vi "SpecAn Capture Screenshot.vi"(0 "VISA In":refnum<visa-resource-name>, 5 "Error In":errorcluster, 6 "Full Screen":bool, 7 "Secured View":bool, 9 "Save Image?":bool) -> (13 "image size":cluster{"Width":u32, "Height":u32}, 14 "VISA Out":refnum<visa-resource-name>, 15 "image data":T1, 16 "Pic":picture, 18 "GIF_PATH":path, 19 "Error Out":errorcluster)   [LabVIEW 2015]
uses:
  <vilib>/picture/picture.llb/imagedata.ctl
  Controls/FGV Action SpecAn Model.ctl
  <vilib>/wsapi/NI_WebServices.lvlib
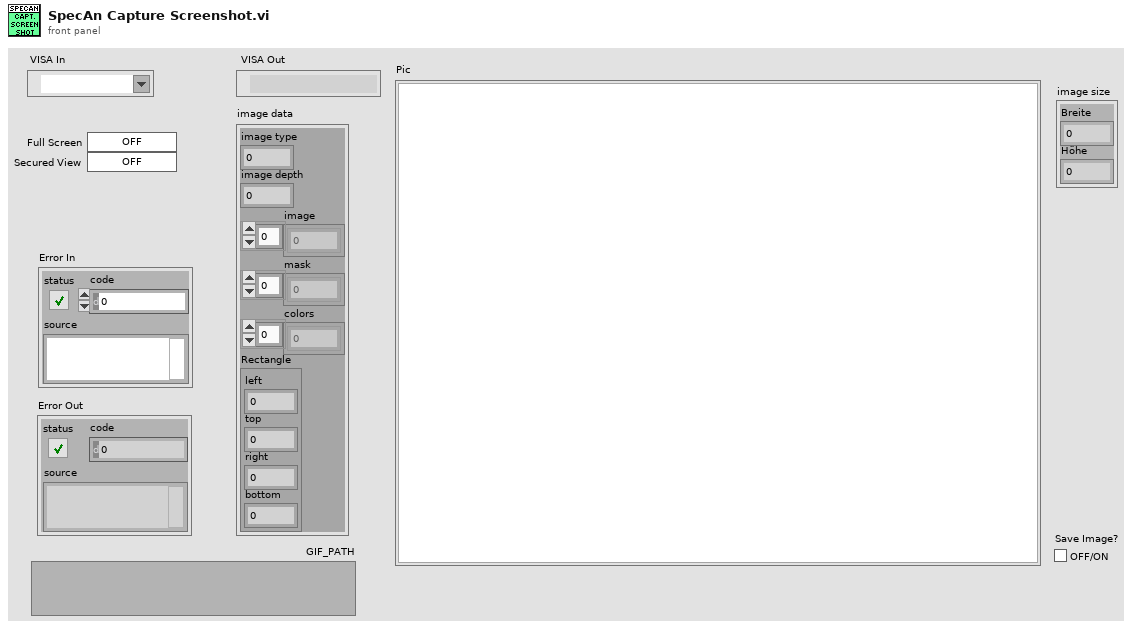
[diagram p1: front panel]
types:
  T1 = typedef "imagedata.ctl" = cluster{"image type":i32, "image depth":i32, "image":u8[], "mask":u8[], "colors":u32[], "Rectangle":cluster{"left":i16, "top":i16, "right":i16, "bottom":i16}}
  T2 = typedef "FGV Action SpecAn Model.ctl" = enum16{"Get", "Set"}
  T3 = typedef "SpecAn Model.ctl" = enum16{"E4440", "N9030"}
  T4 = enum16{"big-endian, network order", "native, host order", "little-endian"}
  T5 = cluster{"left":i16, "top":i16, "right":i16, "bottom":i16}
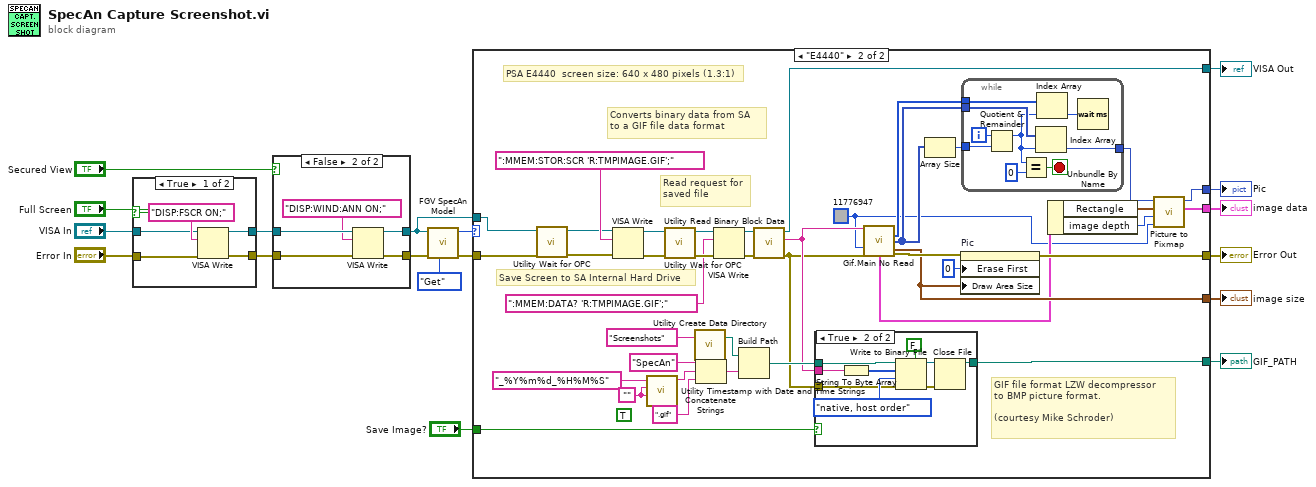
[diagram p0: block diagram]
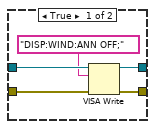
[diagram p2: hidden frame]
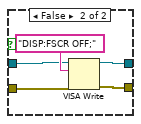
[diagram p3: hidden frame]
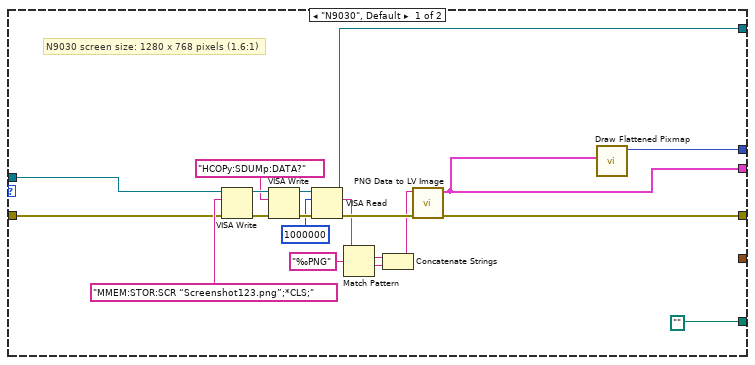
[diagram p4: hidden frame]
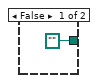
[diagram p5: hidden frame]
diagram:
  n1 = case shown="True" "Full Screen" {
    tunnel: [w22 w27] -> w5
    tunnel: [w21 w26] -> w9
    tunnel: "Error In" -> [w19 w25]
    tunnel: "VISA In" -> [w20 w24]
    frame True {
      n2 = VISA Write(VISA resource name=w20, write buffer="DISP:FSCR ON;", error in (no error)=w19) -> (VISA resource name out=w22:refnum<visa-resource-name>, error out=w21:errorcluster)  [unwired: 1 out]
    }
    frame False {
      n3 = VISA Write(VISA resource name=w24, write buffer="DISP:FSCR OFF;", error in (no error)=w25) -> (VISA resource name out=w27:refnum<visa-resource-name>, error out=w26:errorcluster)  [unwired: 1 out]
    }
  }
  n4 = case shown="False" "Secured View" {
    tunnel: w5 -> [w33 w38]
    tunnel: [w32 w37] -> w3
    tunnel: [w31 w36] -> w4
    tunnel: w9 -> [w29 w34]
    frame True {
      n5 = VISA Write(VISA resource name=w33, write buffer="DISP:WIND:ANN OFF;", error in (no error)=w29) -> (VISA resource name out=w32:refnum<visa-resource-name>, error out=w31:errorcluster)  [unwired: 1 out]
    }
    frame False {
      n6 = VISA Write(VISA resource name=w38, write buffer="DISP:WIND:ANN ON;", error in (no error)=w34) -> (VISA resource name out=w37:refnum<visa-resource-name>, error out=w36:errorcluster)  [unwired: 1 out]
    }
  }
  n7 = call "FGV SpecAn Model.vi"("Action"=FGV_Action_SpecAn_Model."Get", "Error In"=w4, "VISA In"=w3) -> ("Error Out"=w2:errorcluster, "SA Model"=w16:T3)  [unwired: 4 in]
  n8 = case shown="\"E4440\"" w16 {
    tunnel: [w39 w76] -> w14
    tunnel: w2 -> [w48 w60]
    tunnel: w3 -> [w47 w61]
    tunnel: [w46 w91] -> w18
    tunnel: [w43 w63] -> w15
    tunnel: [w42 w62] -> w13
    tunnel: [path "" w71] -> w12
    tunnel: [_ w69] -> w11
    tunnel: "Save Image?" -> [_ w59]
    frame "N9030", Default {
      # "N9030 screen size: 1280 x 768 pixels (1.6:1)"
      n9 = VISA Write(VISA resource name=w47, write buffer="MMEM:STOR:SCR “Screenshot123.png”;*CLS;", error in (no error)=w48) -> (VISA resource name out=w56:refnum<visa-resource-name>, error out=w57:errorcluster)  [unwired: 1 out]
      n10 = VISA Write(VISA resource name=w56, write buffer="HCOPy:SDUMp:DATA?", error in (no error)=w57) -> (VISA resource name out=w53:refnum<visa-resource-name>, error out=w54:errorcluster)  [unwired: 1 out]
      n11 = VISA Read(VISA resource name=w53, byte count=u32 1000000, error in (no error)=w54) -> (VISA resource name out=w46:refnum<visa-resource-name>, read buffer=w44:string, error out=w45:errorcluster)  [unwired: 1 out]
      n12 = Match Pattern(string=w44, regular expression="‰PNG") -> (match substring=w50:string, after substring=w49:string)  [unwired: 1 in, 2 out]
      n13 = Concatenate Strings(w50, w49) -> (w41:string)
      n14 = call <vilib>:"PNG Data to LV Image.vi"("error in (no error)"=w45, "png data"=w41) -> ("error out"=w39:errorcluster, "image data"=w43:T1)  [unwired: 8 in]
      n15 = call <vilib>:"Draw Flattened Pixmap.vi"("image data"=w43) -> ("new picture"=w42:picture)  [unwired: 8 in]
    }
    frame "E4440" {
      (unwired) TRUE
      w82 = ""
      w65 = u32 11776947 ("bgcolor")
      # "PSA E4440  screen size: 640 x 480 pixels (1.3:1)"
      # "GIF file format LZW decompressor\nto BMP picture format.\n\n(courtesy Mike Schroder)"
      # "Converts binary data from SA\nto a GIF file data format"
      # "Read request for\nsaved file"
      # "Save Screen to SA Internal Hard Drive"
      n16 = call "Utility Wait for OPC.vi"("error in (no error)"=w60, "VISA resource name"=w61) -> ("error out"=w89:errorcluster, "VISA resource name out"=w88:refnum<visa-resource-name>)  [unwired: 8 in]
      n17 = VISA Write(VISA resource name=w88, write buffer=":MMEM:STOR:SCR 'R:TMPIMAGE.GIF';", error in (no error)=w89) -> (VISA resource name out=w95:refnum<visa-resource-name>, error out=w93:errorcluster)  [unwired: 1 out]
      n18 = call "Utility Timestamp with Date and Time Strings.vi"("Delimiter (Time)"=w82, "Delimiter (Date)"=w82, "Timestamp Format String"="_%Y%m%d_%H%M%S" ("time format string (%c)")) -> ("Timestamp String"=w80:string)  [unwired: 6 in, 2 out]
      n19 = call "Utility Wait for OPC.vi"("error in (no error)"=w93, "VISA resource name"=w95) -> ("error out"=w94:errorcluster, "VISA resource name out"=w96:refnum<visa-resource-name>)  [unwired: 8 in]
      n20 = call "Utility Create Data Directory.vi"("Folder Name"="Screenshots") -> ("Path"=w84:path)  [unwired: 2 in]
      n21 = Concatenate Strings("SpecAn" ("File Name"), w80, ".gif" ("string")) -> (w79:string)
      n22 = VISA Write(VISA resource name=w96, write buffer=":MMEM:DATA? 'R:TMPIMAGE.GIF';", error in (no error)=w94) -> (VISA resource name out=w98:refnum<visa-resource-name>, error out=w97:errorcluster)  [unwired: 1 out]
      n23 = Build Path(base path=w84, name or relative path=w79) -> (appended path=w77:path)
      n24 = call "Utility Read Binary Block Data.vi"("Error In"=w97, "VISA In"=w98) -> ("Error Out"=w66:errorcluster, "Data"=w74:string, "VISA Out"=w91:refnum<visa-resource-name>)  [unwired: 5 in]
      n25 = case shown="True" w59 {
        tunnel: w77 -> [_ w103]
        tunnel: w74 -> [_ w102]
        tunnel: [path "" w101] -> w71
        tunnel: w66 -> [_ w100]
        frame False {
        }
        frame True {
          n26 = String To Byte Array(string=w102) -> (unsigned byte array=w108:u8[])
          n27 = Write to Binary File(file (use dialog)=w103, data=w108, error in=w100, 5:FALSE ("prepend array or string size? (T)"), 9:T4."native, host order" ("byte order (0:big-endian, network order)")) -> (refnum out=w105:refnum<file>, error out=w106:errorcluster)  [unwired: 1 in, 1 out]
          n28 = Close File(refnum=w105, error in=w106) -> (path=w101:path)  [unwired: 1 out]
        }
      }
      n29 = call "Gif.Main No Read.vi"("bin-string"=w74, "bgcolor"=w65, "error in (no error)"=w66) -> ("time"=w72:u32[], "images out"=w73:picture[], "image data"=w68:T1, "image size"=w69:cluster{"Width":u32, "Height":u32}, "error out"=w75:errorcluster)  [unwired: 8 in]
      n30 = Array Size(array=w73) -> (size(s)=w86:i32)
      n31 = property on="Pic" class="Pict"(error in=w75, "Erase First"=u8 0, "Draw Area Size"=w69) -> (error out=w76:errorcluster)  [unwired: 1 in, 1 out]
      n32 = while {
        tunnel: w72 -> [w114]
        tunnel: w86 -> [w116]
        tunnel: w73 -> [w113]
        tunnel: [w109] -> w70
        i -> [w117]
        stop <- w110 stop-if-true
        n33 = Quotient & Remainder(x=w117, y=w116) -> (x-y*floor(x/y)=w112:i32)  [unwired: 1 out]
        n34 = Equal?(x=w112, y=0) -> (x = y?=w110:bool)
        n35 = Index Array(array=w113, index=w112) -> (element=w109:picture)
        n36 = Index Array(array=w114, index=w112) -> (element=w115:u32)
        n37 = Wait (ms)(milliseconds to wait=w115) -> ()  [unwired: 1 out]
      }
      n38 = Unbundle By Name(w68) -> ("Rectangle"=w67:T5, "image depth"=w64:i32)
      n39 = call <vilib>:"Picture to Pixmap.vi"("Background Color"=w65, "depth"=w64, "rect"=w67, "picture"=w70) -> ("image data"=w63:T1, "new picture"=w62:picture)  [unwired: 6 in]
    }
  }
  "Error Out" <- w14
  "VISA Out" <- w18
  "image data" <- w15
  "Pic" <- w13
  "GIF_PATH" <- w12
  "image size" <- w11
